vi "DataPacker_MIDASMessageHandler.vi"(0 "DataPacker in":refnum<class "DataPacker.lvclass">, 5 "Message":string, 7 "Array":dbl[](array[numeric]), 9 "MIDAS Comm finish time":timestamp, 11 "error in (no error)":errorcluster) -> (4 "DataPacker out":refnum<class "DataPacker.lvclass">, 15 "error out":errorcluster)   [LabVIEW 2018, in "feGEM DataPacker.lvlib" / "DataPacker.lvclass"]
uses:
  DataPacker.lvclass
  DataPacker.lvclass/DataPacker.ctl
  298dbf56-ea75-4091-814e-d94d6c007238.vi
  298dbf56-ea75-4091-814e-d94d6c007238.vi/fceabf22-a343-4e99-aef1-b09667cf9a05.vi
  <vilib>/regexp/Match Regular Expression.xnode
  feGEM DataPacker.lvlib
  <vilib>/Utility/SystemLogging/NI_SystemLogging.lvlib
panel:
  out "Message (HEX)":string
  out "Data":string
  out "JSON Type":string
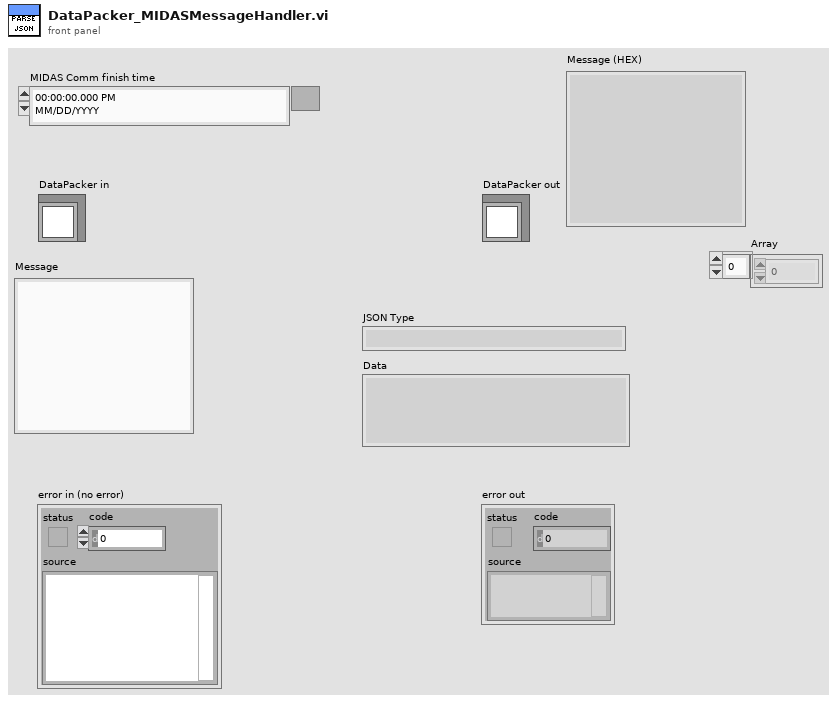
[diagram p1: front panel]
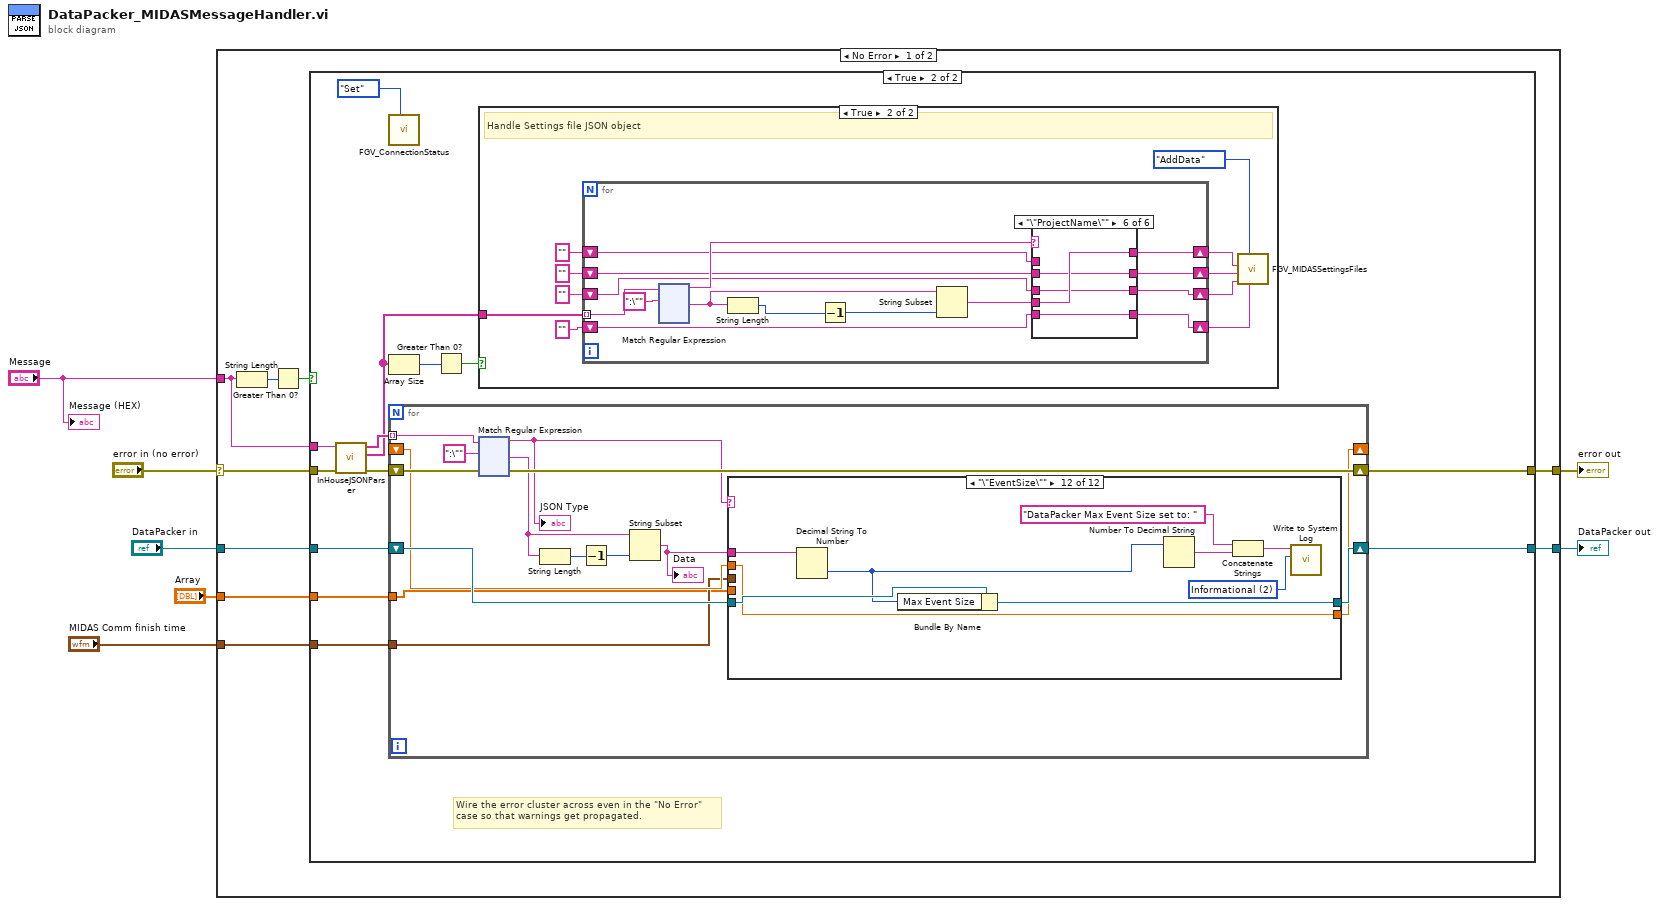
[diagram p0: block diagram]
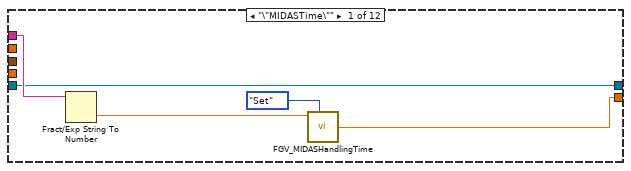
[diagram p9: hidden frame]
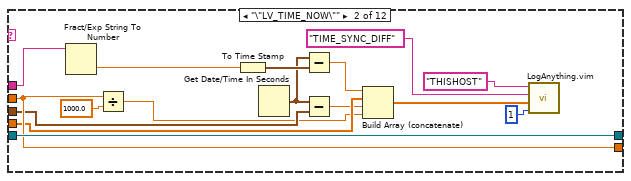
[diagram p10: hidden frame]
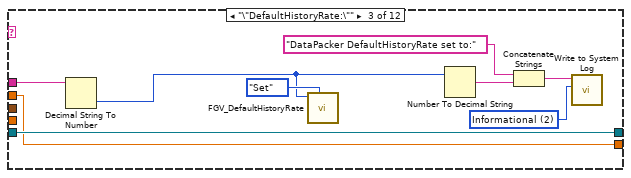
[diagram p11: hidden frame]
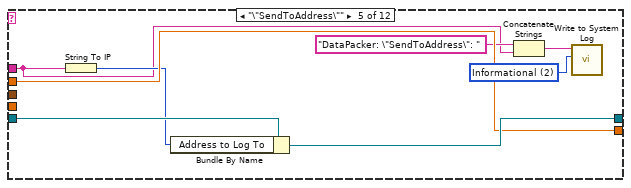
[diagram p13: hidden frame]
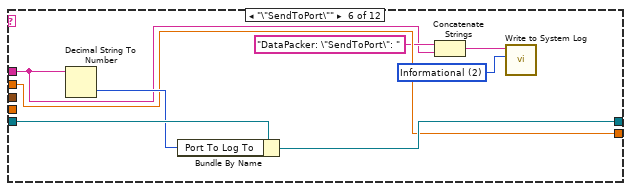
[diagram p14: hidden frame]
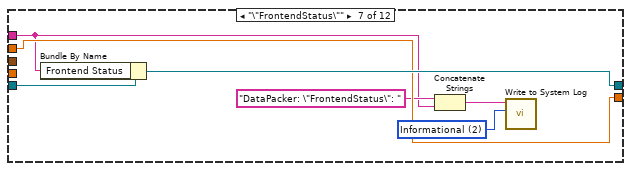
[diagram p15: hidden frame]
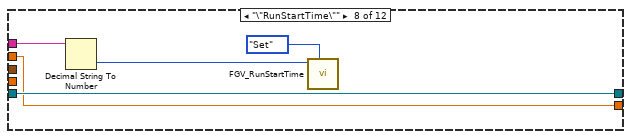
[diagram p16: hidden frame]
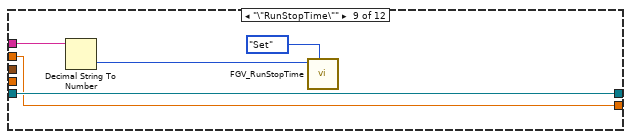
[diagram p17: hidden frame]
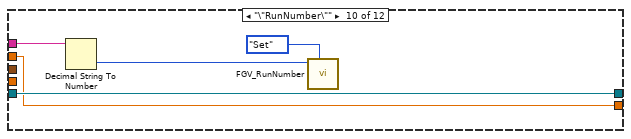
[diagram p18: hidden frame]
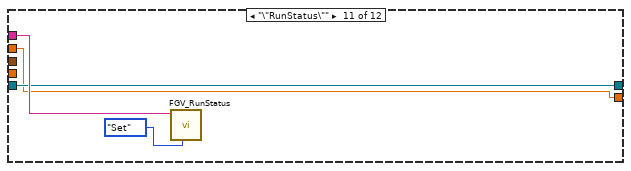
[diagram p19: hidden frame]
diagram:
  n1 = case shown="No Error" "error in (no error)" {
    selector: "error in (no error)" -> [w16 w408]
    tunnel: [w15 w408] -> w6
    tunnel: [w13 w407] -> w3
    tunnel: "DataPacker in" -> [w14 w407]
    tunnel: "Message" -> [w12 _]
    tunnel: "MIDAS Comm finish time" -> [w9 _]
    tunnel: "Array" -> [w8 _]
    frame No Error {
      n2 = String Length(string=w12) -> (length=w11:i32)
      n3 = Greater Than 0?(x=w11) -> (x > 0?=w10:bool)
      n4 = case shown="True" w10 {
        tunnel: w12 -> [_ w26]
        tunnel: w16 -> [w18 w24]
        tunnel: [w18 w31] -> w15
        tunnel: w14 -> [w17 w30]
        tunnel: [w17 w29] -> w13
        tunnel: w9 -> [_ w28]
        tunnel: w8 -> [_ w27]
        frame False {
        }
        frame True {
          # "Wire the error cluster across even in the \"No Error\"\ncase so that warnings get propagated."
          n5 = call "InHouseJSONParser.vi"("error in (no error)"=w24, "feGEM JSON string"=w26) -> ("error out"=w23:errorcluster, "Settings file as array"=w20:string[], "JSON as array"=w25:string[])  [unwired: 7 in]
          n6 = call "FGV_ConnectionStatus.vi"("Enum"=enum16{"Get", "Set"}."Set") -> ()  [unwired: 4 in, 2 out]
          n7 = Array Size(array=w20) -> (size(s)=w22:i32)
          n8 = for {
            tunnel: w25 -> [w209] mode=indexing
            shift-right: [w206] -> w31
            shift-left: w23 -> [w207]
            shift-right: [w204] -> w29
            shift-left: w30 -> [w205]
            shift-right: [w203] -> _
            shift-left: _ -> [w202]
            tunnel: w28 -> [w201]
            tunnel: w27 -> [w200]
            n9 = xnode "Match Regular Expression"("input string"=w209, "regular expression"=":\"", "error in"=w207) -> ("before match"=w199:string, "after match"=w198:string, "error out"=w206:errorcluster)  [unwired: 3 in, 2 out]
            "JSON Type" <- w199
            n10 = String Length(string=w198) -> (length=w197:i32)
            n11 = Decrement(x=w197) -> (x-1=w196:i32)
            n12 = String Subset(string=w198, length (rest)=w196) -> (substring=w195:string)  [unwired: 1 in]
            "Data" <- w195
            n13 = case shown="\"\\\"EventSize\\\"\"" w199 {
              tunnel: w195 -> [w327 w340 w352 _ w358 w366 w374 w383 w388 w391 w396 w406]
              tunnel: w205 -> [w325 w342 w351 w355 w363 w371 w378 w380 w385 w390 w395 w405]
              tunnel: [w325 w342 w351 w355 w362 w370 w377 w380 w385 w390 w395 w404] -> w204
              tunnel: [w324 w336 w350 w354 w361 w368 w376 w379 w384 w389 w394 w403] -> w203
              tunnel: w202 -> [_ w336 w350 w354 w361 w368 w376 w379 w384 w389 w394 w403]
              tunnel: w201 -> [_ w331 _ _ _ _ _ _ _ _ _ _]
              tunnel: w200 -> [_ w335 _ _ _ _ _ _ _ _ _ _]
              frame "\"MIDASTime\"" {
                n14 = Fract/Exp String To Number(string=w327) -> (number=w328:dbl)  [unwired: 3 in, 1 out]
                n15 = call "FGV_MIDASHandlingTime.vi"("Midas Handling Time"=w328, "Enum"=enum16{"Set", "GetLast", "GetAverage"}."Set") -> ("Midas Handling Time"=w324:dbl)  [unwired: 3 in]
              }
              frame "\"LV_TIME_NOW\"" {
                n16 = Fract/Exp String To Number(string=w340) -> (number=w339:dbl)  [unwired: 3 in, 1 out]
                n17 = Divide(x=w336, y=1000.0) -> (x/y=w329:dbl)
                n18 = To Time Stamp(1:w339) -> (0:w333:timestamp)
                n19 = Get Date/Time In Seconds() -> (seconds since 1Jan1904=w332:timestamp)
                n20 = Subtract(x=w332, y=w333) -> (x-y=w334:dbl)
                n21 = Subtract(x=w332, y=w331) -> (x-y=w330:dbl)
                n22 = Build Array (concatenate)(w334, w335, w330, w329) -> (w341:dbl[])
                n23 = call "LogAnything.vim"("Period to update history plots (seconds)\nUnset (65535) = Use MIDAS default in ODB\n0 = Record but do not put in histories"=u16 1 ("Period to update history plots (seconds)\nUnset (65535) = Use MIDAS default in ODB\n0 = Record but do not put in histories"), "Array"=w341, "Variable Name"="TIME_SYNC_DIFF", "Category"="THISHOST") -> ()  [unwired: 6 in, 2 out]
              }
              frame "\"DefaultHistoryRate:\"" {
                w345 = 2 items=["Error", "Warning", "Informational"] ("severity")
                n24 = Decimal String To Number(string=w352) -> (number=w347:i32)  [unwired: 2 in, 1 out]
                n25 = call "FGV_DefaultHistoryRate.vi"("Default History Rate"=w347, "Enum"=enum16{"Set", "Get"}."Set") -> ()  [unwired: 3 in, 1 out]
                n26 = Number To Decimal String(number=w347) -> (decimal integer string=w346:string)  [unwired: 1 in]
                n27 = Concatenate Strings("DataPacker DefaultHistoryRate set to:" ("message"), w346) -> (w348:string)
                n28 = call <vilib>:"Write to System Log.vi"("severity"=w345, "message"=w348) -> ()  [unwired: 9 in, 1 out]
              }
              frame "False", Default {
              }
              frame "\"SendToAddress\"" {
                w356 = 2 items=["Error", "Warning", "Informational"] ("severity")
                n29 = String To IP(1:w358) -> (0:w360:u32)
                n30 = Bundle By Name(cluster=w363, "Address to Log To"=w360) -> (w362:refnum<class "DataPacker.lvclass">)
                n31 = Concatenate Strings("DataPacker: \"SendToAddress\": " ("message"), w358) -> (w357:string)
                n32 = call <vilib>:"Write to System Log.vi"("severity"=w356, "message"=w357) -> ()  [unwired: 9 in, 1 out]
              }
              frame "\"SendToPort\"" {
                w364 = 2 items=["Error", "Warning", "Informational"] ("severity")
                n33 = Decimal String To Number(string=w366) -> (number=w369:i32)  [unwired: 2 in, 1 out]
                n34 = Bundle By Name(cluster=w371, "Port To Log To"=w369) -> (w370:refnum<class "DataPacker.lvclass">)
                n35 = Concatenate Strings("DataPacker: \"SendToPort\": " ("message"), w366) -> (w365:string)
                n36 = call <vilib>:"Write to System Log.vi"("severity"=w364, "message"=w365) -> ()  [unwired: 9 in, 1 out]
              }
              frame "\"FrontendStatus\"" {
                w372 = 2 items=["Error", "Warning", "Informational"] ("severity")
                n37 = Bundle By Name(cluster=w378, "Frontend Status"=w374) -> (w377:refnum<class "DataPacker.lvclass">)
                n38 = Concatenate Strings("DataPacker: \"FrontendStatus\": " ("message"), w374) -> (w373:string)
                n39 = call <vilib>:"Write to System Log.vi"("severity"=w372, "message"=w373) -> ()  [unwired: 9 in, 1 out]
              }
              frame "\"RunStartTime\"" {
                n40 = Decimal String To Number(string=w383) -> (number=w382:i32)  [unwired: 2 in, 1 out]
                n41 = call "FGV_RunStartTime.vi"("Run Start Time"=w382, "Enum"=enum16{"Set", "Get"}."Set") -> ()  [unwired: 3 in, 2 out]
              }
              frame "\"RunStopTime\"" {
                n42 = Decimal String To Number(string=w388) -> (number=w387:i32)  [unwired: 2 in, 1 out]
                n43 = call "FGV_RunStopTime.vi"("Run Stop Time"=w387, "Enum"=enum16{"Set", "Get"}."Set") -> ()  [unwired: 3 in, 2 out]
              }
              frame "\"RunNumber\"" {
                n44 = Decimal String To Number(string=w391) -> (number=w393:i32)  [unwired: 2 in, 1 out]
                n45 = call "FGV_RunNumber.vi"("Run Number"=w393, "Enum"=enum16{"Set", "Get"}."Set") -> ()  [unwired: 3 in, 1 out]
              }
              frame "\"RunStatus\"" {
                n46 = call "FGV_RunStatus.vi"("Run Status"=w396, "Enum"=enum16{"Set", "Get"}."Set") -> ()  [unwired: 3 in, 1 out]
              }
              frame "\"EventSize\"" {
                w398 = 2 items=["Error", "Warning", "Informational"] ("severity")
                n47 = Decimal String To Number(string=w406) -> (number=w400:i32)  [unwired: 2 in, 1 out]
                n48 = Bundle By Name(cluster=w405, "Max Event Size"=w400) -> (w404:refnum<class "DataPacker.lvclass">)
                n49 = Number To Decimal String(number=w400) -> (decimal integer string=w399:string)  [unwired: 1 in]
                n50 = Concatenate Strings("DataPacker Max Event Size set to: " ("message"), w399) -> (w401:string)
                n51 = call <vilib>:"Write to System Log.vi"("severity"=w398, "message"=w401) -> ()  [unwired: 9 in, 1 out]
              }
            }
          }
          n52 = Greater Than 0?(x=w22) -> (x > 0?=w21:bool)
          n53 = case shown="True" w21 {
            tunnel: w20 -> [_ w41]
            frame False {
            }
            frame True {
              # "Handle Settings file JSON object"
              n54 = for {
                tunnel: w41 -> [w55] mode=indexing
                shift-right: [w49] -> w39
                shift-left: "" ("after match") -> [w43]
                shift-right: [w48] -> w38
                shift-left: "" ("after match") -> [w44]
                shift-right: [w47] -> w37
                shift-left: "" ("after match") -> [w45]
                shift-right: [w46] -> w36
                shift-left: "" ("after match") -> [w42]
                n55 = xnode "Match Regular Expression"("input string"=w55, "regular expression"=":\"") -> ("before match"=w54:string, "after match"=w51:string)  [unwired: 4 in, 3 out]
                n56 = String Length(string=w51) -> (length=w53:i32)
                n57 = Decrement(x=w53) -> (x-1=w52:i32)
                n58 = String Subset(string=w51, length (rest)=w52) -> (substring=w50:string)  [unwired: 1 in]
                n59 = case shown="\"\\\"ProjectName\\\"\"" w54 {
                  tunnel: w50 -> [_ w178 _ w186 w190 w194]
                  tunnel: [w174 w177 w182 w185 w187 w194] -> w49
                  tunnel: [w173 w178 w181 w184 w188 w193] -> w48
                  tunnel: [w172 w176 w180 w186 w189 w192] -> w47
                  tunnel: [w171 w175 w179 w183 w190 w191] -> w46
                  tunnel: w45 -> [w172 w176 w180 _ w189 w192]
                  tunnel: w44 -> [w173 _ w181 w184 w188 w193]
                  tunnel: w43 -> [w174 w177 w182 w185 w187 _]
                  tunnel: w42 -> [w171 w175 w179 w183 _ w191]
                  frame "False", Default {
                  }
                  frame "\"Filename\"" {
                  }
                  frame "\"UNIXTIME\"" {
                  }
                  frame "\"MD5\"" {
                  }
                  frame "\"base64data\"" {
                  }
                  frame "\"ProjectName\"" {
                  }
                }
              }
              n60 = call "FGV_MIDASSettingsFiles.vi"("BinaryData"=w36, "Enum"=enum16{"AddData", "Set", "Get"}."AddData", "MD5 (optional)"=w37, "FileName"=w38, "ProjectName"=w39) -> ()  [unwired: 4 in, 3 out]
            }
          }
        }
      }
    }
    frame Error {
    }
  }
  "error out" <- w6
  "DataPacker out" <- w3
  "Message (HEX)" <- "Message"
